vi "test moxa.vi"() -> ()   [LabVIEW 2016]
uses:
  <vilib>/Instr/_visa.llb/VISA Configure Serial Port (Instr).vi
panel:
  out "stop 2":bool
  in  "write 2":bool
  in  "Write":bool
  out "Serial Settings:Number of Bytes at Serial Port 2":u32
  out "Serial Settings:Number of Bytes at Serial Port":u32
  out "read buffer 2":string
  in  "write buffer 2":string
  out "read buffer":string
  in  "write buffer":string
  out "loop":i32
  in  "VISA resource name 2":refnum<visa-resource-name>="COM8"
  in  "baud rate (9600) 2":u32=115200
  in  "stop":bool
  out "error out":errorcluster
  in  "error in (no error)":errorcluster
  in  "baud rate (9600)":u32=115200
  in  "VISA resource name":refnum<visa-resource-name>="COM7"
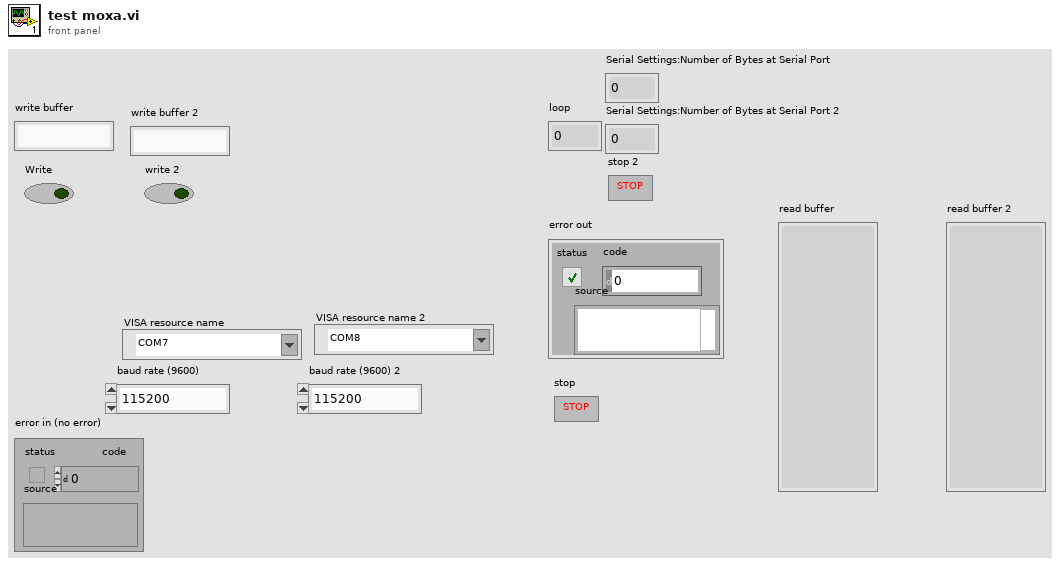
[diagram p1: front panel]
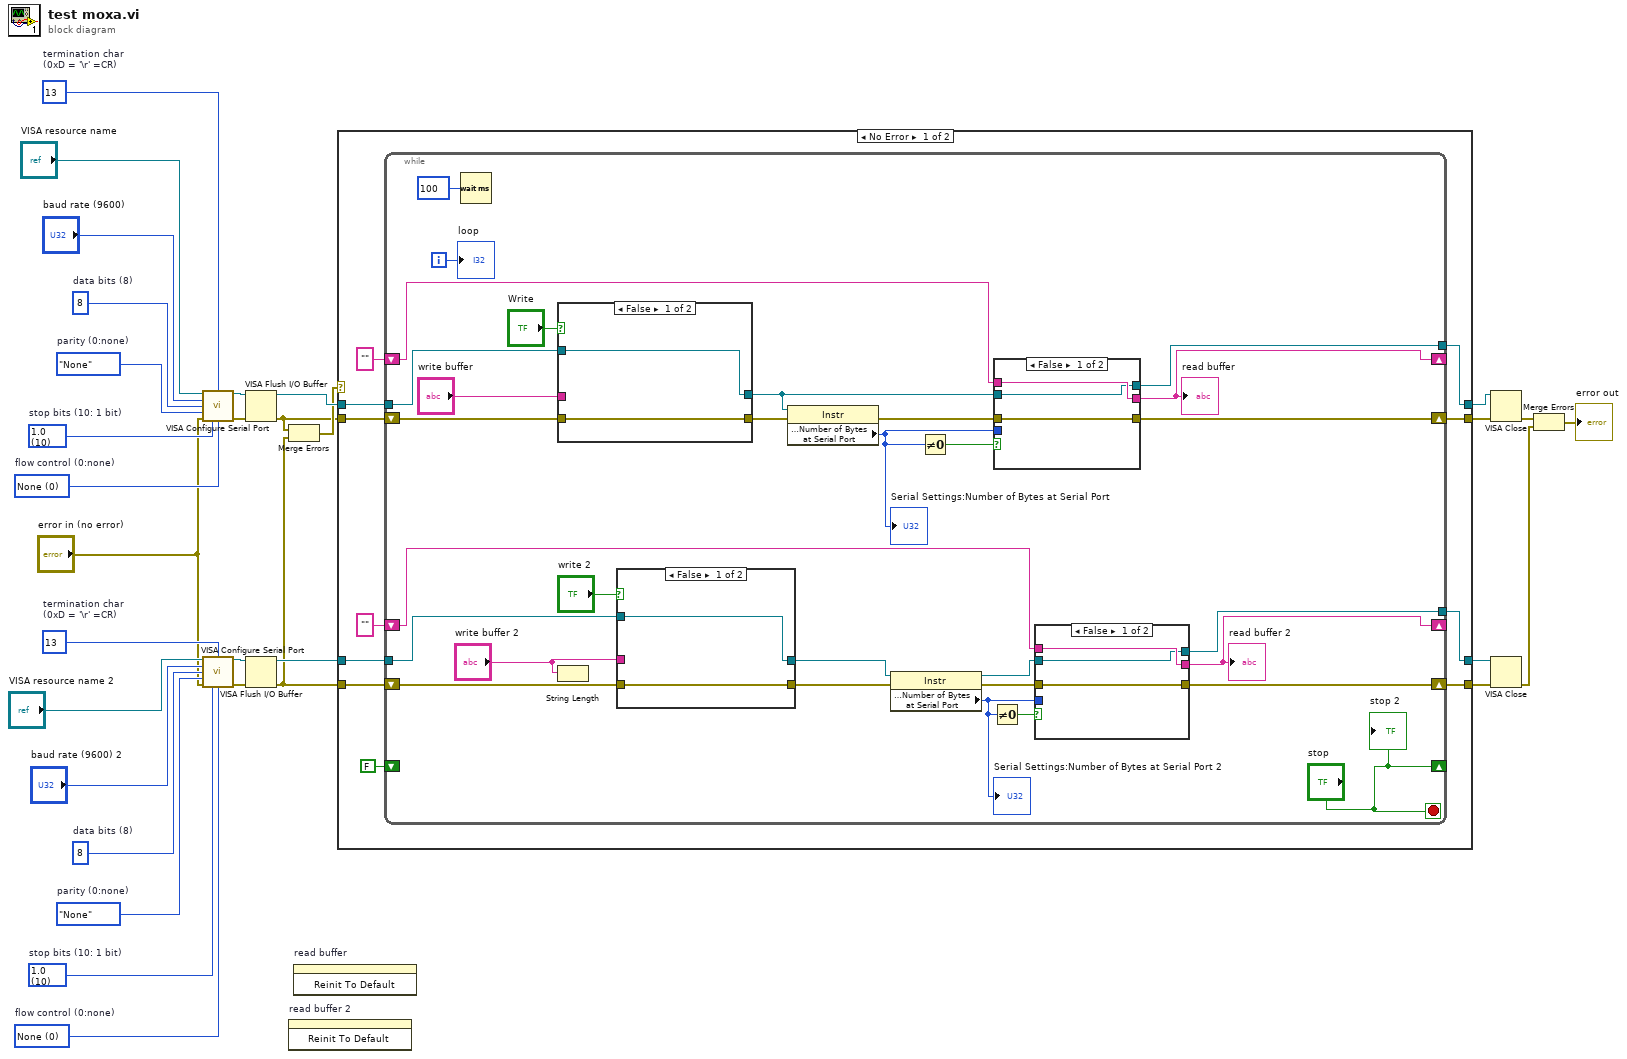
[diagram p0: block diagram]
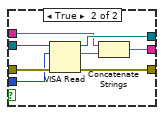
[diagram p2: hidden frame]
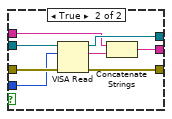
[diagram p3: hidden frame]
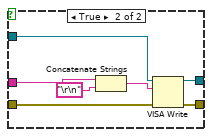
[diagram p4: hidden frame]
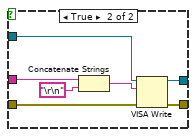
[diagram p5: hidden frame]
diagram:
  w21 = u8 13  # termination char (0xD = '\r' =CR)
  w18 = u16 0 items=["None", "XON/XOFF", "RTS/CTS", "XON/XOFF & RTS/CTS", "DTR/DSR", "XON/XOFF & DTR/DSR"]  # flow control (0:none)
  w17 = u16 10 items=["1.0"=10, "1.5"=15, "2.0"=20]  # stop bits (10: 1 bit)
  w16 = enum16{"None", "Odd", "Even", "Mark", "Space"}."None"  # parity (0:none)
  w15 = u16 8  # data bits (8)
  w23 = u8 13  # termination char (0xD = '\r' =CR)
  w26 = u16 0 items=["None", "XON/XOFF", "RTS/CTS", "XON/XOFF & RTS/CTS", "DTR/DSR", "XON/XOFF & DTR/DSR"]  # flow control (0:none)
  w27 = u16 10 items=["1.0"=10, "1.5"=15, "2.0"=20]  # stop bits (10: 1 bit)
  w28 = enum16{"None", "Odd", "Even", "Mark", "Space"}."None"  # parity (0:none)
  w29 = u16 8  # data bits (8)
  n1 = call-poly "VISA Configure Serial Port"("VISA resource name"="VISA resource name", "termination char\n(0xA = '\\n' = LF)"=w23, "baud rate (9600)"="baud rate (9600)", "data bits (8)"=w29, "parity (0:none)"=w28, "error in (no error)"="error in (no error)", "stop bits (10: 1 bit)"=w27, "flow control (0:none)"=w26) -> ("VISA resource name out"=w24:refnum<visa-resource-name>, "error out"=w25:errorcluster)  [unwired: 6 in]
  n2 = call-poly "VISA Configure Serial Port"("VISA resource name"="VISA resource name 2", "termination char\n(0xA = '\\n' = LF)"=w21, "baud rate (9600)"="baud rate (9600) 2", "data bits (8)"=w15, "parity (0:none)"=w16, "error in (no error)"="error in (no error)", "stop bits (10: 1 bit)"=w17, "flow control (0:none)"=w18) -> ("VISA resource name out"=w20:refnum<visa-resource-name>, "error out"=w19:errorcluster)  [unwired: 6 in]
  n3 = VISA Flush I/O Buffer(VISA resource name=w24, error in (no error)=w25) -> (VISA resource name out=w22:refnum<visa-resource-name>, error out=w2:errorcluster)  [unwired: 1 in]
  n4 = VISA Flush I/O Buffer(VISA resource name=w20, error in (no error)=w19) -> (VISA resource name out=w12:refnum<visa-resource-name>, error out=w1:errorcluster)  [unwired: 1 in]
  n5 = Merge Errors(w2, w1) -> (w3:errorcluster)
  n6 = invoke on="read buffer 2" class="Str" method="Reinit To Default"() -> ()  [unwired: 3 in, 3 out]
  n7 = invoke on="read buffer" class="Str" method="Reinit To Default"() -> ()  [unwired: 3 in, 3 out]
  n8 = case shown="No Error" w3 {
    tunnel: w2 -> [w42 w115]
    tunnel: w22 -> [w41 w116]
    tunnel: w12 -> [w40 w114]
    tunnel: w1 -> [w39 w113]
    tunnel: [w38 w113] -> w11
    tunnel: [w37 w114] -> w10
    tunnel: [w36 w115] -> w9
    tunnel: [w35 w116] -> w8
    frame No Error {
      n9 = while {
        tunnel: w41 -> [w71]
        shift-right: [w70] -> w36
        shift-left: w42 -> [w72]
        tunnel: w40 -> [w66]
        shift-right: [w67] -> w38
        shift-left: w39 -> [w68]
        tunnel: [w69] -> w35
        tunnel: [w63] -> w37
        shift-right: [w54] -> _
        shift-left: "" ("read buffer") -> [w55]
        shift-right: [w52] -> _
        shift-left: "" -> [w53]
        shift-right: ["stop"] -> _
        shift-left: FALSE ("stop") -> [_]
        i -> [w65]
        stop <- "stop" stop-if-true
        n10 = Wait (ms)(milliseconds to wait=u32 100) -> ()  [unwired: 1 out]
        n11 = case shown="False" "Write" {
          tunnel: w72 -> [w96 w103]
          tunnel: w71 -> [w95 w102]
          tunnel: [w95 w101] -> w62
          tunnel: [w96 w100] -> w60
          tunnel: "write buffer" -> [_ w99]
          frame False {
          }
          frame True {
            n12 = Concatenate Strings(w99, "\r\n") -> (w98:string)
            n13 = VISA Write(VISA resource name=w102, write buffer=w98, error in (no error)=w103) -> (VISA resource name out=w101:refnum<visa-resource-name>, error out=w100:errorcluster)  [unwired: 1 out]
          }
        }
        n14 = String Length(string="write buffer 2") -> ()  [unwired: 1 out]
        n15 = case shown="False" "write 2" {
          tunnel: w68 -> [w105 w112]
          tunnel: w66 -> [w104 w111]
          tunnel: "write buffer 2" -> [_ w110]
          tunnel: [w105 w109] -> w59
          tunnel: [w104 w108] -> w57
          frame False {
          }
          frame True {
            n16 = Concatenate Strings(w110, "\r\n") -> (w107:string)
            n17 = VISA Write(VISA resource name=w111, write buffer=w107, error in (no error)=w112) -> (VISA resource name out=w108:refnum<visa-resource-name>, error out=w109:errorcluster)  [unwired: 1 out]
          }
        }
        n18 = property class="Instr"(reference=w62, error in=w60) -> (error out=w61:errorcluster, "Serial Settings:Number of Bytes at Serial Port"=w49:u32)  [unwired: 1 out]
        "Serial Settings:Number of Bytes at Serial Port" <- w49
        n19 = property class="Instr"(reference=w57, error in=w59) -> (reference out=w56:refnum<visa-resource-name>, error out=w58:errorcluster, "Serial Settings:Number of Bytes at Serial Port"=w48:u32)
        "Serial Settings:Number of Bytes at Serial Port 2" <- w48
        n20 = Not Equal To 0?(x=w49) -> (x != 0?=w46:bool)
        n21 = Not Equal To 0?(x=w48) -> (x != 0?=w47:bool)
        n22 = case shown="False" w46 {
          tunnel: [w75 w83] -> w70
          tunnel: [w73 w82] -> w69
          tunnel: w62 -> [w73 w81]
          tunnel: w61 -> [w75 w80]
          tunnel: w55 -> [w74 w79]
          tunnel: [w74 w77] -> w54
          tunnel: w49 -> [_ w76]
          frame False {
          }
          frame True {
            n23 = VISA Read(VISA resource name=w81, byte count=w76, error in (no error)=w80) -> (VISA resource name out=w82:refnum<visa-resource-name>, read buffer=w78:string, error out=w83:errorcluster)  [unwired: 1 out]
            n24 = Concatenate Strings(w79, w78) -> (w77:string)
          }
        }
        "read buffer" <- w54
        n25 = case shown="False" w47 {
          tunnel: [w85 w94] -> w67
          tunnel: [w84 w93] -> w63
          tunnel: w58 -> [w85 w92]
          tunnel: w56 -> [w84 w91]
          tunnel: w53 -> [w86 w90]
          tunnel: [w86 w88] -> w52
          tunnel: w48 -> [_ w87]
          frame False {
          }
          frame True {
            n26 = VISA Read(VISA resource name=w91, byte count=w87, error in (no error)=w92) -> (VISA resource name out=w93:refnum<visa-resource-name>, read buffer=w89:string, error out=w94:errorcluster)  [unwired: 1 out]
            n27 = Concatenate Strings(w90, w89) -> (w88:string)
          }
        }
        "read buffer 2" <- w52
        "loop" <- w65
        "stop 2" <- "stop"
      }
    }
    frame Error {
    }
  }
  n28 = VISA Close(VISA resource name=w8, error in (no error)=w9) -> (error out=w6:errorcluster)
  n29 = VISA Close(VISA resource name=w10, error in (no error)=w11) -> (error out=w7:errorcluster)
  n30 = Merge Errors(w6, w7) -> (→"error out":errorcluster)
